vi "relay_init.vi"(4 "VISA resource in":refnum<visa-resource-name>="COM12") -> (1 "relay session out":T1={"VISA resource out"="COM12", "error out"={"status"=FALSE, "code"=0, "source"=""}})   [LabVIEW 2010]
uses:
  <vilib>/Instr/_visa.llb/VISA Configure Serial Port (Instr).vi
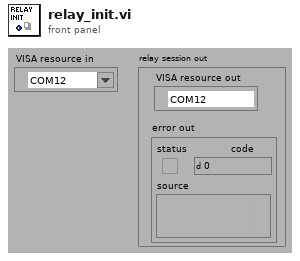
[diagram p1: front panel]
types:
  T1 = cluster{"VISA resource out":refnum<visa-resource-name>, "error out":errorcluster}
  T2 = cluster{"baud rate (9600)":u32, "data bits (8)":u16, "parity (0:none)":enum16{"None", "Odd", "Even", "Mark", "Space"}, "stop bits (10: 1 bit)":u16, "flow control (0:none)":u16, "timeout (10sec)":u32, "termination char\n(0xA = '\\n' = LF) ":u8, "Enable Termination\nChar (T)":bool}
  T3 = cluster{"VISA resource name out":refnum<visa-resource-name>, "error out":errorcluster}
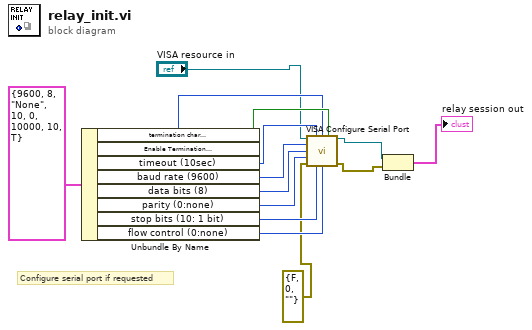
[diagram p0: block diagram]
diagram:
  # "Configure serial port if requested"
  n1 = Unbundle By Name(T2 {"baud rate (9600)"=9600, "data bits (8)"=8, "parity (0:none)"=enum."None", "stop bits (10: 1 bit)"=10, "flow control (0:none)"=0, "timeout (10sec)"=10000, "termination char\n(0xA = '\\n' = LF) "=10, "Enable Termination\nChar (T)"=TRUE} ("Port Configuration")) -> ("termination char\n(0xA = '\\n' = LF)"=w6:u8, "Enable Termination\nChar (T)"=w7:bool, "timeout (10sec)"=w8:u32, "baud rate (9600)"=w13:u32, "data bits (8)"=w12:u16, "parity (0:none)"=w11:enum16{"None", "Odd", "Even", "Mark", "Space"}, "stop bits (10: 1 bit)"=w10:u16, "flow control (0:none)"=w9:u16)
  n2 = call-poly "VISA Configure Serial Port"("VISA resource name"="VISA resource in", "timeout (10sec)"=w8, "termination char\n(0xA = '\\n' = LF)"=w6, "Enable Termination\nChar (T)"=w7, "baud rate (9600)"=w13, "data bits (8)"=w12, "parity (0:none)"=w11, "error in (no error)"=errorcluster {"status"=FALSE, "code"=0, "source"=""} ("error out"), "stop bits (10: 1 bit)"=w10, "flow control (0:none)"=w9) -> ("VISA resource name out"=w4:refnum<visa-resource-name>, "error out"=w3:errorcluster)  [unwired: 4 in]
  n3 = Bundle("VISA resource name out"=w4, "error out"=w3) -> (→"relay session out":T3)  [unwired: 1 in]
